vi "James.vi"(0 "Initial Case":enum16{"Theta", "Arc"}(ring), 5 "Drive Case":enum16{"FOD", "ROD"}(ring), 7 "Cyborg":dbl[](array[numeric]), 9 "Logitech":dbl[](array[numeric]), 11 "gyro":dbl format="%#_13g") -> (4 "A":dbl, 6 "B":dbl, 8 "R":dbl)   [LabVIEW 2014]
panel:
  in  "beta":dbl format="%#_13g"
  in  "alpha":dbl format="%#_13g"
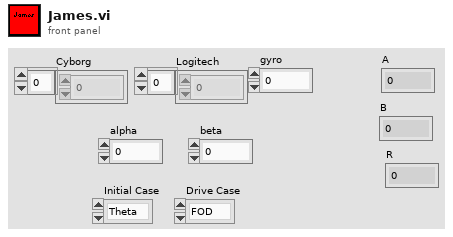
[diagram p1: front panel]
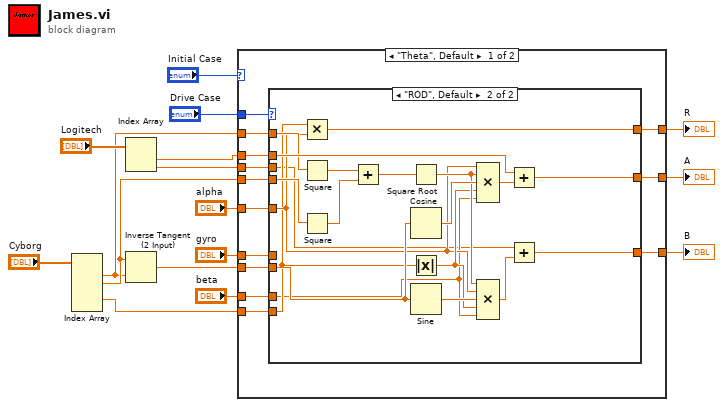
[diagram p0: block diagram]
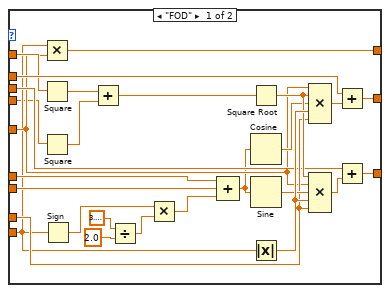
[diagram p2: hidden frame]
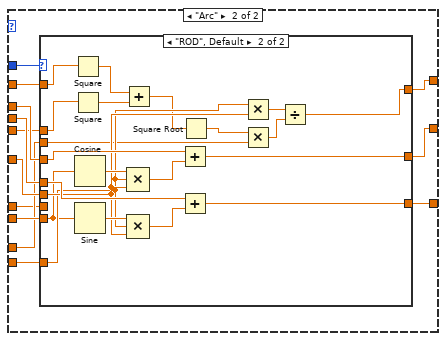
[diagram p3: hidden frame]
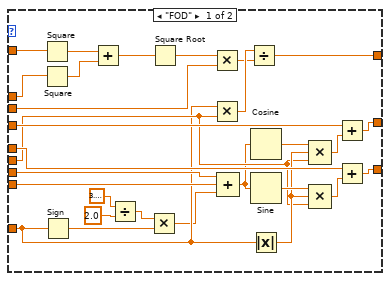
[diagram p4: hidden frame]
diagram:
  n1 = Index Array(array="Cyborg") -> (element #1=w5:dbl, element #2=w6:dbl, element #4=w11:dbl)  [unwired: 5 in, 2 out]
  n2 = Index Array(array="Logitech") -> (element #1=w9:dbl, element #2=w2:dbl)  [unwired: 2 in]
  n3 = Inverse Tangent (2 Input)(1:w5, 2:w6) -> (0:w8:dbl)
  n4 = case shown="\"Theta\", Default" "Initial Case" {
    tunnel: "Drive Case" -> [w29 w89]
    tunnel: w11 -> [w28 w87]
    tunnel: "alpha" -> [w27 w85]
    tunnel: [w26 w78] -> w13
    tunnel: w9 -> [w25 w88]
    tunnel: w8 -> [w24 w86]
    tunnel: "beta" -> [w23 w81]
    tunnel: w6 -> [w22 w79]
    tunnel: w5 -> [w21 w80]
    tunnel: [w20 w84] -> w4
    tunnel: [w19 w82] -> w3
    tunnel: w2 -> [w18 w83]
    tunnel: "gyro" -> [w17 w77]
    frame "Theta", Default {
      n5 = case shown="\"ROD\", Default" w29 {
        tunnel: w28 -> [w31 w61]
        tunnel: w27 -> [w40 w62]
        tunnel: [w43 w76] -> w26
        tunnel: w25 -> [w46 w75]
        tunnel: w24 -> [w34 w65]
        tunnel: w23 -> [w47 w60]
        tunnel: w22 -> [w30 w72]
        tunnel: w21 -> [w44 w71]
        tunnel: [w41 w59] -> w20
        tunnel: [w42 w58] -> w19
        tunnel: w18 -> [w45 w57]
        tunnel: w17 -> [w32 _]
        frame "FOD" {
          n6 = Multiply(x=w31, y=w40) -> (x*y=w43:dbl)
          n7 = Square(x=w44) -> (x^2=w51:dbl)
          n8 = Square(x=w30) -> (x^2=w50:dbl)
          n9 = Sign(1:w31) -> (0:w39:dbl)
          n10 = Add(x=w51, y=w50) -> (x+y=w52:dbl)
          n11 = Divide(x=3.141592653589793, y=2.0) -> (x/y=w36:dbl)
          n12 = Multiply(x=w39, y=w36) -> (x*y=w35:dbl)
          n13 = Compound Arithmetic op=ADD(w32, w34, w35) -> (w33:dbl)
          n14 = Square Root(x=w52) -> (sqrt(x)=w55:dbl)
          n15 = Cosine(x=w33) -> (cos(x)=w48:dbl)
          n16 = Sine(x=w33) -> (sin(x)=w53:dbl)
          n17 = Absolute Value(x=w31) -> (abs(x)=w56:dbl)
          n18 = Compound Arithmetic op=MULTIPLY(w40, w55, w48, w56, w47) -> (w49:dbl)
          n19 = Compound Arithmetic op=MULTIPLY(w55, w40, w53, w56, w47) -> (w54:dbl)
          n20 = Add(x=w46, y=w49) -> (x+y=w41:dbl)
          n21 = Add(x=w45, y=w54) -> (x+y=w42:dbl)
        }
        frame "ROD", Default {
          n22 = Multiply(x=w61, y=w62) -> (x*y=w76:dbl)
          n23 = Square(x=w71) -> (x^2=w69:dbl)
          n24 = Square(x=w72) -> (x^2=w70:dbl)
          n25 = Add(x=w69, y=w70) -> (x+y=w68:dbl)
          n26 = Square Root(x=w68) -> (sqrt(x)=w64:dbl)
          n27 = Cosine(x=w65) -> (cos(x)=w74:dbl)
          n28 = Absolute Value(x=w61) -> (abs(x)=w63:dbl)
          n29 = Sine(x=w65) -> (sin(x)=w67:dbl)
          n30 = Compound Arithmetic op=MULTIPLY(w62, w64, w74, w63, w60) -> (w73:dbl)
          n31 = Compound Arithmetic op=MULTIPLY(w64, w62, w67, w63, w60) -> (w66:dbl)
          n32 = Add(x=w75, y=w73) -> (x+y=w59:dbl)
          n33 = Add(x=w57, y=w66) -> (x+y=w58:dbl)
        }
      }
    }
    frame "Arc" {
      n34 = case shown="\"ROD\", Default" w89 {
        tunnel: w88 -> [w105 w139]
        tunnel: w87 -> [w95 w129]
        tunnel: w86 -> [w97 w122]
        tunnel: w85 -> [w100 w130]
        tunnel: [w108 w135] -> w84
        tunnel: w83 -> [w104 w133]
        tunnel: [w106 w132] -> w82
        tunnel: w81 -> [w90 w128]
        tunnel: w80 -> [w103 w125]
        tunnel: w79 -> [w102 w123]
        tunnel: [w107 w120] -> w78
        tunnel: w77 -> [w99 _]
        frame "FOD" {
          n35 = Square(x=w103) -> (x^2=w112:dbl)
          n36 = Square(x=w102) -> (x^2=w111:dbl)
          n37 = Sign(1:w95) -> (0:w96:dbl)
          n38 = Add(x=w112, y=w111) -> (x+y=w109:dbl)
          n39 = Divide(x=3.141592653589793, y=2.0) -> (x/y=w92:dbl)
          n40 = Multiply(x=w92, y=w96) -> (x*y=w91:dbl)
          n41 = Square Root(x=w109) -> (sqrt(x)=w113:dbl)
          n42 = Multiply(x=w113, y=w90) -> (x*y=w110:dbl)
          n43 = Multiply(x=w95, y=w100) -> (x*y=w114:dbl)
          n44 = Compound Arithmetic op=ADD(w99, w97, w91) -> (w98:dbl)
          n45 = Divide(x=w114, y=w110) -> (x/y=w107:dbl)
          n46 = Cosine(x=w98) -> (cos(x)=w117:dbl)
          n47 = Sine(x=w98) -> (sin(x)=w116:dbl)
          n48 = Absolute Value(x=w95) -> (abs(x)=w101:dbl)
          n49 = Compound Arithmetic op=MULTIPLY(w117, w101, w100) -> (w118:dbl)
          n50 = Compound Arithmetic op=MULTIPLY(w116, w101, w100) -> (w115:dbl)
          n51 = Add(x=w105, y=w118) -> (x+y=w108:dbl)
          n52 = Add(x=w104, y=w115) -> (x+y=w106:dbl)
        }
        frame "ROD", Default {
          n53 = Square(x=w125) -> (x^2=w126:dbl)
          n54 = Square(x=w123) -> (x^2=w124:dbl)
          n55 = Cosine(x=w122) -> (cos(x)=w137:dbl)
          n56 = Sine(x=w122) -> (sin(x)=w136:dbl)
          n57 = Add(x=w126, y=w124) -> (x+y=w119:dbl)
          n58 = Compound Arithmetic op=MULTIPLY(w137, w129, w130) -> (w138:dbl)
          n59 = Compound Arithmetic op=MULTIPLY(w136, w129, w130) -> (w134:dbl)
          n60 = Add(x=w139, y=w138) -> (x+y=w135:dbl)
          n61 = Add(x=w133, y=w134) -> (x+y=w132:dbl)
          n62 = Square Root(x=w119) -> (sqrt(x)=w127:dbl)
          n63 = Multiply(x=w129, y=w130) -> (x*y=w131:dbl)
          n64 = Multiply(x=w127, y=w128) -> (x*y=w121:dbl)
          n65 = Divide(x=w131, y=w121) -> (x/y=w120:dbl)
        }
      }
    }
  }
  "R" <- w13
  "A" <- w4
  "B" <- w3
